vi "pdw to raw PDW.vi"(8 "erorr in":errorcluster, 10 "Fs":i32, 11 "PDW":T1(array[cluster])) -> (0 "erorr out":errorcluster, 2 "lfm lost":bool, 3 "Array":u64[](array[numeric]))   [LabVIEW 2021]
uses:
  pdw.ctl
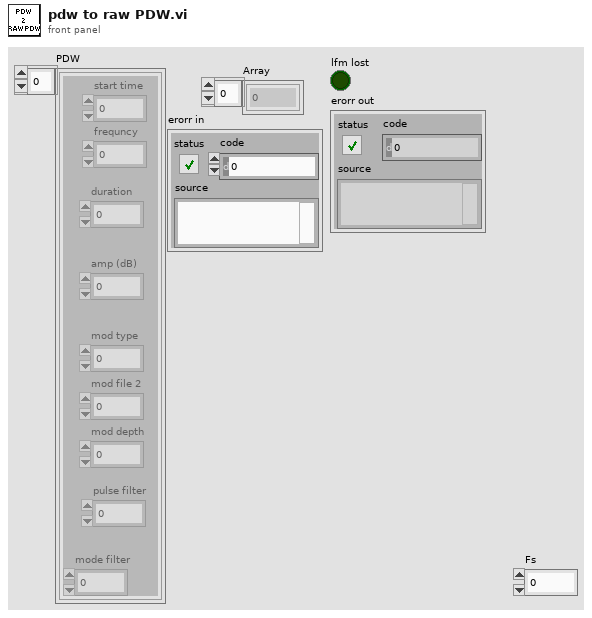
[diagram p1: front panel]
types:
  T1 = cluster{"start time":dbl, "frequncy":dbl, "duration":dbl, "amp (dB)":dbl, "mod type":u8, "mod file 2":u8, "mod depth":dbl, "pulse filter":u16, "mode filter ":u16}[]
  T2 = typedef "pdw.ctl" = cluster{"PW":u32, "frequency shift":fxp<+/-,48,0>, "amp":fxp<+/-,18,1>, "mode type":u8, "mode file":u8, "mode depth":u32, "filter rate_pulse":u16, "filter rate bpsk":u16}
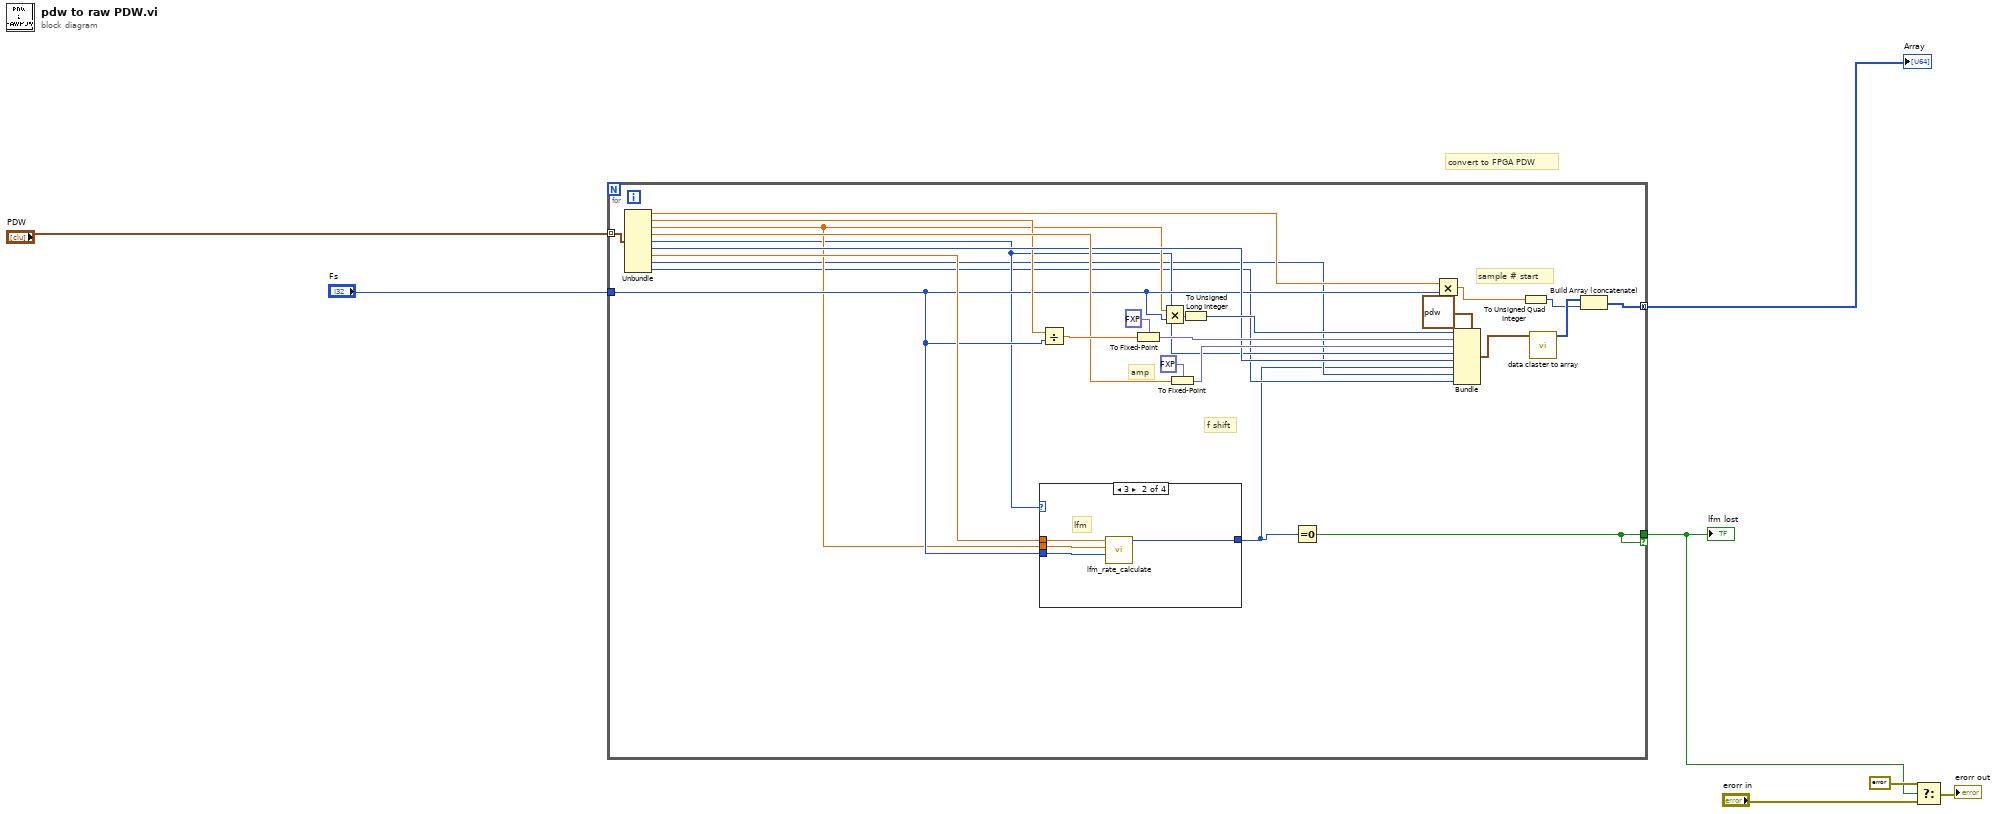
[diagram p0: block diagram]
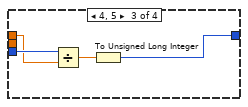
[diagram p3: hidden frame]
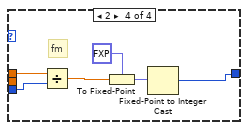
[diagram p4: hidden frame]
diagram:
  # "convert to FPGA PDW"
  n1 = for {
    tunnel: "PDW" -> [w33] mode=indexing
    tunnel: [w19] -> w5 mode=concatenating
    tunnel: "Fs" -> [w14]
    tunnel: [w8] -> w2 if=w8
    # "amp"
    # "f shift"
    # "sample # start"
    n2 = Unbundle(w33) -> ("start time"=w32:dbl, "frequncy"=w15:dbl, "duration"=w13:dbl, "amp (dB)"=w26:dbl, "mod type"=w12:u8, "mod file 2"=w17:u8, "mod depth"=w16:dbl, "pulse filter"=w11:u16, "mode filter"=w10:u16)
    n3 = case shown="3" w12 {
      tunnel: [_ w34 w38 w42] -> w9
      tunnel: w14 -> [_ w37 w41 w46]
      tunnel: w16 -> [_ w36 w40 w47]
      tunnel: w13 -> [_ w35 _ _]
      frame Default {
        # "not fm mode"
      }
      frame 3 {
        # "lfm"
        n4 = call "lfm_rate_calculate.vi"("fs"=w37, "pw"=w35, "f span"=w36) -> ("integer (fxp cast)"=w34:u32)  [unwired: 8 in]
      }
      frame 4, 5 {
        n5 = Divide(x=w41, y=w40) -> (x/y=w39:dbl)
        n6 = To Unsigned Long Integer(number=w39) -> (unsigned 32bit integer=w38:u32)
      }
      frame 2 {
        # "fm"
        n7 = Divide(x=w47, y=w46) -> (x/y=w43:dbl)
        n8 = To Fixed-Point(fixed-point type=fxp<+,32,-16> 0.0, number=w43) -> (fixed-point=w45:fxp<+,32,-16>)
        n9 = Fixed-Point to Integer Cast(1:w45) -> (0:w42:u32)
      }
    }
    n10 = Divide(x=w15, y=w14) -> (x/y=w30:dbl)
    n11 = To Fixed-Point(fixed-point type=fxp<+/-,48,0> 0.0 ("frequency shift"), number=w30) -> (fixed-point=w28:fxp<+/-,48,0>)
    n12 = Multiply(x=w13, y=w14) -> (x*y=w27:dbl)
    n13 = To Fixed-Point(fixed-point type=fxp<+/-,18,1> 0.0 ("I"), number=w26) -> (fixed-point=w24:fxp<+/-,18,1>)
    n14 = To Unsigned Long Integer(number=w27) -> (unsigned 32bit integer=w18:u32)
    n15 = Equal To 0?(x=w9) -> (x = 0?=w8:bool)
    n16 = Multiply(x=w32, y=w14) -> (x*y=w31:dbl)
    n17 = Bundle(cluster=T2 {"PW"=0, "frequency shift"=0.0, "amp"=0.0, "mode type"=0, "mode file"=0, "mode depth"=0, "filter rate_pulse"=0, "filter rate bpsk"=0} ("Cluster"), "PW"=w18, "frequency shift"=w28, "amp"=w24, "mode type"=w12, "mode file"=w17, "mode depth"=w9, "filter rate_pulse"=w11, "filter rate bpsk"=w10) -> (w20:T2)
    n18 = To Unsigned Quad Integer(1:w31) -> (0:w22:u64)
    n19 = call "data claster to array.vi"("Cluster"=w20) -> ("Array"=w23:u64[])  [unwired: 10 in]
    n20 = Build Array (concatenate)(w23, w22) -> (w19:u64[])
  }
  "Array" <- w5
  "lfm lost" <- w2
  n21 = Select(t=errorcluster {"status"=TRUE, "code"=5432, "source"="The LFM value lost, pls take higher value for it"} ("error out"), s=w2, f="erorr in") -> (s? t:f=→"erorr out":errorcluster)
